vi "Main Tclk.vi"() -> ()   [LabVIEW 2018] (continued)
            n6787 = local read "Faraday Cup < Milling current"() -> (w2106:bool)
            n6788 = local read "FIB"() -> (w2105:bool)
            n6789 = local read "Email Alert Recipients"() -> (w2110:string[])
            n6790 = local read "Mail server"() -> (w2111:string)
            n6791 = local read "Hardware Configuration"() -> (w2113:T25)
            n6792 = local read "Email Log Files"() -> (w2108:path)
            n6793 = Unbundle By Name(w2113) -> ("Machine ID"=w2112:string)
            n6794 = Compound Arithmetic op=AND(w2105, w2106) -> (w2107:bool)
            n6795 = call "Email alert.vi"("Email log file path"=w2108, "Send email"=w2107, "Machine ID"=w2112, "Mail server"=w2111, "Alarm message"="Faraday cup current < Milling current", "Recipents"=w2110) -> ()  [unwired: 6 in]
            n6796 = case shown="True" w2107 {
              frame False {
              }
              frame True {
                n6797 = stacked-sequence {
                  frame #0 {
                    n6798 = Wait (ms)(milliseconds to wait=u32 200) -> ()  [unwired: 1 out]
                  }
                  frame #1 {
                    n6799 = local write "Faraday Cup < Milling current"(FALSE ("E-mail test")) -> ()
                  }
                }
              }
            }
          }
          frame #6 {
            n6800 = local read "SEM Status"() -> (w2122:T12)
            n6801 = Unbundle By Name(w2122) -> ("SEM Spec. I (nA)"=w2119:sgl)
            n6802 = local read "FIB"() -> (w2118:bool)
            n6803 = local read "SEM Spec. I spike"() -> (w2117:bool)
            n6804 = local read "Email Alert Recipients"() -> (w2127:string[])
            n6805 = local read "Mail server"() -> (w2128:string)
            n6806 = local read "Hardware Configuration"() -> (w2130:T25)
            n6807 = local read "Email Log Files"() -> (w2126:path)
            n6808 = Format Into String(format string="%#g", w2119) -> (resulting string=w2120:string)  [unwired: 2 in, 1 out]
            n6809 = Compound Arithmetic op=AND(w2118, w2117) -> (w2116:bool)
            n6810 = Unbundle By Name(w2130) -> ("Machine ID"=w2129:string)
            n6811 = Concatenate Strings("SEM specimen current spiked to " ("Alarm message"), w2120, " nA" ("Alarm message")) -> (w2124:string)
            n6812 = call "Email alert.vi"("Email log file path"=w2126, "Send email"=w2116, "Machine ID"=w2129, "Mail server"=w2128, "Alarm message"=w2124, "Recipents"=w2127) -> ()  [unwired: 6 in]
            n6813 = case shown="True" w2116 {
              frame False {
              }
              frame True {
                n6814 = stacked-sequence {
                  frame #0 {
                    n6815 = Wait (ms)(milliseconds to wait=u32 200) -> ()  [unwired: 1 out]
                  }
                  frame #1 {
                    n6816 = local write "SEM Spec. I spike"(FALSE ("E-mail test")) -> ()
                  }
                }
              }
            }
          }
          frame #7 {
            n6817 = local read "Milling Z voltage (V)"() -> (w2136:sgl)
            n6818 = local read "FIB"() -> (w2135:bool)
            n6819 = local read "Milling Z voltage spike"() -> (w2134:bool)
            n6820 = local read "Email Alert Recipients"() -> (w2143:string[])
            n6821 = local read "Mail server"() -> (w2144:string)
            n6822 = local read "Hardware Configuration"() -> (w2146:T25)
            n6823 = local read "Email Log Files"() -> (w2142:path)
            n6824 = Format Into String(format string="%#g", w2136) -> (resulting string=w2137:string)  [unwired: 2 in, 1 out]
            n6825 = Unbundle By Name(w2146) -> ("Machine ID"=w2145:string)
            n6826 = Compound Arithmetic op=AND(w2135, w2134) -> (w2133:bool)
            n6827 = Concatenate Strings("Milling Z voltage spiked to " ("Alarm message"), w2137, " V" ("Alarm message")) -> (w2140:string)
            n6828 = call "Email alert.vi"("Email log file path"=w2142, "Send email"=w2133, "Machine ID"=w2145, "Mail server"=w2144, "Alarm message"=w2140, "Recipents"=w2143) -> ()  [unwired: 6 in]
            n6829 = case shown="True" w2133 {
              frame False {
              }
              frame True {
                n6830 = stacked-sequence {
                  frame #0 {
                    n6831 = Wait (ms)(milliseconds to wait=u32 200) -> ()  [unwired: 1 out]
                  }
                  frame #1 {
                    n6832 = local write "Milling Z voltage spike"(FALSE ("E-mail test")) -> ()
                  }
                }
              }
            }
          }
          frame #8 {
            n6833 = local read "Alert Settings"() -> (w2153:T36)
            n6834 = local read "FIB"() -> (w2149:bool)
            n6835 = Unbundle By Name(w2153) -> ("EHT off alarm"=w2152:bool)
            n6836 = local read "EHT off"() -> (w2154:bool)
            n6837 = local read "Email Alert Recipients"() -> (w2156:string[])
            n6838 = local read "Mail server"() -> (w2157:string)
            n6839 = local read "Hardware Configuration"() -> (w2159:T25)
            n6840 = local read "Email Log Files"() -> (w2150:path)
            n6841 = Compound Arithmetic op=AND(w2149, w2152, w2154) -> (w2151:bool)
            n6842 = Unbundle By Name(w2159) -> ("Machine ID"=w2158:string)
            n6843 = call "Email alert.vi"("Email log file path"=w2150, "Send email"=w2151, "Machine ID"=w2158, "Mail server"=w2157, "Alarm message"="EHT was off", "Recipents"=w2156) -> ()  [unwired: 6 in]
            n6844 = case shown="True" w2151 {
              frame False {
              }
              frame True {
                n6845 = stacked-sequence {
                  frame #0 {
                    n6846 = Wait (ms)(milliseconds to wait=u32 200) -> ()  [unwired: 1 out]
                  }
                  frame #1 {
                    n6847 = local write "EHT off"(FALSE ("E-mail test")) -> ()
                  }
                }
              }
            }
          }
          frame #9 {
            n6848 = local read "Alert Settings"() -> (w2166:T36)
            n6849 = local read "FIB"() -> (w2162:bool)
            n6850 = local read "Det A over scale"() -> (w2164:bool)
            n6851 = local read "Email Alert Recipients"() -> (w2169:string[])
            n6852 = local read "Mail server"() -> (w2170:string)
            n6853 = local read "Hardware Configuration"() -> (w2172:T25)
            n6854 = local read "Email Log Files"() -> (w2167:path)
            n6855 = Unbundle By Name(w2166) -> ("Detector over scale warning"=w2165:bool)
            n6856 = Unbundle By Name(w2172) -> ("Machine ID"=w2171:string)
            n6857 = Compound Arithmetic op=AND(w2162, w2165, w2164) -> (w2163:bool)
            n6858 = call "Email alert.vi"("Email log file path"=w2167, "Send email"=w2163, "Machine ID"=w2171, "Mail server"=w2170, "Alarm message"="Detector A over scale", "Recipents"=w2169) -> ()  [unwired: 6 in]
            n6859 = case shown="True" w2163 {
              frame False {
              }
              frame True {
                n6860 = stacked-sequence {
                  frame #0 {
                    n6861 = Wait (ms)(milliseconds to wait=u32 200) -> ()  [unwired: 1 out]
                  }
                  frame #1 {
                    n6862 = local write "Det A over scale"(FALSE ("E-mail test")) -> ()
                  }
                }
              }
            }
          }
          frame #10 {
            n6863 = local read "Alert Settings"() -> (w2179:T36)
            n6864 = local read "FIB"() -> (w2175:bool)
            n6865 = local read "Email Alert Recipients"() -> (w2182:string[])
            n6866 = local read "Mail server"() -> (w2183:string)
            n6867 = local read "Hardware Configuration"() -> (w2185:T25)
            n6868 = local read "Email Log Files"() -> (w2180:path)
            n6869 = local read "Det B over scale"() -> (w2177:bool)
            n6870 = Unbundle By Name(w2179) -> ("Detector over scale warning"=w2178:bool)
            n6871 = Unbundle By Name(w2185) -> ("Machine ID"=w2184:string)
            n6872 = Compound Arithmetic op=AND(w2175, w2178, w2177) -> (w2176:bool)
            n6873 = call "Email alert.vi"("Email log file path"=w2180, "Send email"=w2176, "Machine ID"=w2184, "Mail server"=w2183, "Alarm message"="Detector B over scale", "Recipents"=w2182) -> ()  [unwired: 6 in]
            n6874 = case shown="True" w2176 {
              frame False {
              }
              frame True {
                n6875 = stacked-sequence {
                  frame #0 {
                    n6876 = Wait (ms)(milliseconds to wait=u32 200) -> ()  [unwired: 1 out]
                  }
                  frame #1 {
                    n6877 = local write "Det B over scale"(FALSE ("E-mail test")) -> ()
                  }
                }
              }
            }
          }
          frame #11 {
            n6878 = local read "Alert Settings"() -> (w2190:T36)
            n6879 = local read "3D image paused active"() -> (w2193:bool)
            n6880 = local read "3D image paused armed"() -> (w2191:bool)
            n6881 = local read "Hardware Configuration"() -> (w2198:T25)
            n6882 = local read "Email Log Files"() -> (w2188:path)
            n6883 = Unbundle By Name(w2190) -> ("3D imaging paused alarm"=w2189:bool)
            n6884 = Unbundle By Name(w2198) -> ("Machine ID"=w2194:string)
            n6885 = case shown="True" w2193 {
              frame False {
              }
              frame True {
                n6886 = stacked-sequence {
                  frame #0 {
                    n6887 = Wait (ms)(milliseconds to wait=u32 500) -> ()  [unwired: 1 out]
                  }
                  frame #1 {
                    w2200 = FALSE ("3D image paused active bypass")
                    n6888 = local write "3D image paused active"(w2200) -> ()
                    "3D image paused armed" <- w2200
                  }
                }
              }
            }
            n6889 = Compound Arithmetic op=AND(w2193, w2191, w2189) -> (w2192:bool)
            n6890 = call "Email alert.vi"("Email log file path"=w2188, "Send email"=w2192, "Machine ID"=w2194, "Mail server"="Mail server", "Alarm message"="3D imaging paused", "Recipents"="Email Alert Recipients") -> ()  [unwired: 6 in]
          }
          frame #12 {
            n6891 = local read "Alert Settings"() -> (w2206:T36)
            n6892 = local read "Email Alert Recipients"() -> (w2210:string[])
            n6893 = local read "API timeout"() -> (w2201:bool)
            n6894 = local read "SW error warning active"() -> (w2203:bool)
            n6895 = local read "SW error warning armed"() -> (w2207:bool)
            n6896 = local read "Mail server"() -> (w2211:string)
            n6897 = local read "Hardware Configuration"() -> (w2213:T25)
            n6898 = local read "Email Log Files"() -> (w2204:path)
            n6899 = Unbundle By Name(w2206) -> ("SW error warning"=w2205:bool)
            n6900 = Or(x=w2201, y=w2203) -> (x .or. y?=w2202:bool)
            n6901 = Unbundle By Name(w2213) -> ("Machine ID"=w2212:string)
            n6902 = Compound Arithmetic op=AND(w2202, w2207, w2205) -> (w2208:bool)
            n6903 = call "Email alert.vi"("Email log file path"=w2204, "Send email"=w2208, "Machine ID"=w2212, "Mail server"=w2211, "Alarm message"="Software timeout error", "Recipents"=w2210) -> ()  [unwired: 6 in]
            n6904 = case shown="True" w2202 {
              frame False {
              }
              frame True {
                n6905 = stacked-sequence {
                  frame #0 {
                    n6906 = Wait (ms)(milliseconds to wait=u32 500) -> ()  [unwired: 1 out]
                  }
                  frame #1 {
                    w2215 = FALSE ("3D image paused active bypass")
                    n6907 = local write "SW error warning active"(w2215) -> ()
                    "SW error warning armed" <- w2215
                  }
                }
              }
            }
          }
          frame #13 {
            n6908 = local read "SEM shutter failed active"() -> (w2224:bool)
            n6909 = local read "SEM shutter warning armed"() -> (w2225:bool)
            n6910 = local read "Email Alert Recipients"() -> (w2227:string[])
            n6911 = local read "Mail server"() -> (w2228:string)
            n6912 = local read "Hardware Configuration"() -> (w2230:T25)
            n6913 = local read "Email Log Files"() -> (w2223:path)
            n6914 = local read "Fail #"() -> (w2216:u8)
            n6915 = Greater Than 0?(x=w2216) -> (x > 0?=w2217:bool)
            n6916 = Format Into String(format string="%#g", w2216) -> (resulting string=w2220:string)  [unwired: 2 in, 1 out]
            n6917 = Concatenate Strings("SEM shutter failed " ("Alarm message"), w2220, " times" ("Alarm message")) -> (w2218:string)
            n6918 = Unbundle By Name(w2230) -> ("Machine ID"=w2229:string)
            n6919 = Compound Arithmetic op=AND(w2224, w2225, w2217) -> (w2226:bool)
            n6920 = call "Email alert.vi"("Email log file path"=w2223, "Send email"=w2226, "Machine ID"=w2229, "Mail server"=w2228, "Alarm message"=w2218, "Recipents"=w2227) -> ()  [unwired: 6 in]
            n6921 = case shown="True" w2224 {
              frame False {
              }
              frame True {
                n6922 = stacked-sequence {
                  frame #0 {
                    n6923 = Wait (ms)(milliseconds to wait=u32 500) -> ()  [unwired: 1 out]
                  }
                  frame #1 {
                    w2232 = FALSE ("3D image paused active bypass")
                    n6924 = local write "SEM shutter failed active"(w2232) -> ()
                    "SEM shutter warning armed" <- w2232
                  }
                }
              }
            }
          }
          frame #14 {
            n6925 = local read "Machine Type"() -> (w2233:u8)
            n6926 = case shown="2" w2233 {
              tunnel: [w2249 w2263] -> w2236
              frame 0, Default {
                w2244 = "%#g" ("format string")
                n6927 = local read "Actual Reheat Parameters"() -> (w2257:T1)
                n6928 = local read "HV Data Output"() -> (w2248:T18)
                n6929 = Unbundle By Name(w2248) -> ("Tip Lifetime (hr)"=w2247:sgl)
                n6930 = Unbundle By Name(w2257) -> ("Filament I (A)"=w2256:sgl, "Reheat time (s)"=w2255:sgl)
                n6931 = Format Into String(format string=w2244, w2256) -> (resulting string=w2253:string)  [unwired: 2 in, 1 out]
                n6932 = Format Into String(format string="%d", w2247) -> (resulting string=w2245:string)  [unwired: 2 in, 1 out]
                n6933 = Format Into String(format string=w2244, w2255) -> (resulting string=w2251:string)  [unwired: 2 in, 1 out]
                n6934 = Concatenate Strings("FIB lifetime = " ("Alarm message"), w2245, " hr, FIB reheat started, " ("Alarm message"), w2253, " A for " ("string"), w2251, " s" ("string")) -> (w2249:string)
              }
              frame 2 {
                n6935 = local read "Capella HV Data Output"() -> (w2262:T17)
                n6936 = Unbundle By Name(w2262) -> ("Tip Lifetime (uAhr)"=w2261:sgl)
                n6937 = Format Into String(format string="%d", w2261) -> (resulting string=w2259:string)  [unwired: 2 in, 1 out]
                n6938 = Concatenate Strings("FIB lifetime = " ("Alarm message"), w2259, " uAhr, FIB reheat started" ("Alarm message")) -> (w2263:string)
              }
            }
            n6939 = local read "Mail server"() -> (w2240:string)
            n6940 = local read "Hardware Configuration"() -> (w2242:T25)
            n6941 = local read "Send reheat start email"() -> (w2234:bool)
            n6942 = local read "Reheat warning armed"() -> (w2237:bool)
            n6943 = local read "Email Alert Recipients"() -> (w2239:string[])
            n6944 = Unbundle By Name(w2242) -> ("Machine ID"=w2241:string)
            n6945 = Compound Arithmetic op=AND(w2234, w2237) -> (w2238:bool)
            n6946 = local read "Email Log Files"() -> (w2235:path)
            n6947 = call "Email alert.vi"("Email log file path"=w2235, "Send email"=w2238, "Machine ID"=w2241, "Mail server"=w2240, "Alarm message"=w2236, "Recipents"=w2239) -> ()  [unwired: 6 in]
            n6948 = case shown="True" w2234 {
              frame False {
              }
              frame True {
                n6949 = stacked-sequence {
                  frame #0 {
                    n6950 = Wait (ms)(milliseconds to wait=u32 500) -> ()  [unwired: 1 out]
                  }
                  frame #1 {
                    w2266 = FALSE ("3D image paused active bypass")
                    n6951 = local write "Send reheat start email"(w2266) -> ()
                    "Reheat warning armed" <- w2266
                  }
                }
              }
            }
          }
          frame #15 {
            n6952 = local read "Start Reheat"() -> (w2278:bool)
            n6953 = local read "Reheat warning armed"() -> (w2277:bool)
            n6954 = local read "Reheat completed"() -> (w2274:bool)
            n6955 = local read "Machine Type"() -> (w2267:u8)
            n6956 = case shown="2" w2267 {
              tunnel: [w2297 w2319] -> w2271
              tunnel: [w2291 w2316] -> w2268
              frame 0, Default {
                w2283 = "%5.1f" ("format string")
                w2285 = "%#g" ("format string")
                n6957 = local read "Reheat Output"() -> (w2305:T21)
                n6958 = local read "HV Data Output"() -> (w2292:T18)
                n6959 = Unbundle By Name(w2305) -> ("Initial emission (uA)"=w2304:sgl, "Initial suppressor (V)"=w2303:sgl, "V/I Slope"=w2296:sgl, "Reheat Success"=w2291:bool)
                n6960 = Unbundle By Name(w2292) -> ("Suppressor (V)"=w2290:sgl, "Emission (uA)"=w2288:sgl)
                n6961 = Format Into String(format string=w2283, w2304) -> (resulting string=w2301:string)  [unwired: 2 in, 1 out]
                n6962 = Format Into String(format string=w2283, w2296) -> (resulting string=w2295:string)  [unwired: 2 in, 1 out]
                n6963 = Format Into String(format string=w2285, w2290) -> (resulting string=w2289:string)  [unwired: 2 in, 1 out]
                n6964 = Format Into String(format string=w2285, w2303) -> (resulting string=w2299:string)  [unwired: 2 in, 1 out]
                n6965 = Format Into String(format string="%3.1f", w2288) -> (resulting string=w2287:string)  [unwired: 2 in, 1 out]
                n6966 = Concatenate Strings("FIB reheat completed successfully, initial emission: " ("Alarm message"), w2301, " uA @ suppressor = " ("element"), w2299, " V, V/I slope = " ("element"), w2295, ", suppressor = " ("string"), w2289, " V @ " ("string"), w2287, " uA emission " ("string")) -> (w2297:string)
              }
              frame 2 {
                w2306 = "%3.1f" ("format string")
                n6967 = local read "Capella HV Data Output"() -> (w2317:T17)
                n6968 = local read "Reheat Output"() -> (w2320:T21)
                n6969 = Unbundle By Name(w2320) -> ("Reheat Success"=w2316:bool)
                n6970 = Unbundle By Name(w2317) -> ("Suppressor (V)"=w2315:sgl, "Emission Actual (uA)"=w2313:sgl)
                n6971 = local read "FIB V/I slope"() -> (w2308:sgl)
                n6972 = Format Into String(format string=w2306, w2308) -> (resulting string=w2307:string)  [unwired: 2 in, 1 out]
                n6973 = Format Into String(format string="%5.1f", w2315) -> (resulting string=w2314:string)  [unwired: 2 in, 1 out]
                n6974 = Format Into String(format string=w2306, w2313) -> (resulting string=w2312:string)  [unwired: 2 in, 1 out]
                n6975 = Concatenate Strings("FIB reheat completed successfully, suppressor =  " ("Alarm message"), w2314, " V @ " ("string"), w2312, " uA emission, V/I slope =  " ("string"), w2307) -> (w2319:string)
              }
            }
            n6976 = local read "Mail server"() -> (w2280:string)
            n6977 = local read "Hardware Configuration"() -> (w2282:T25)
            n6978 = Not(x=w2278) -> (.not. x?=w2275:bool)
            n6979 = Not(x=w2277) -> (.not. x?=w2276:bool)
            n6980 = Unbundle By Name(w2282) -> ("Machine ID"=w2281:string)
            n6981 = Compound Arithmetic op=AND(w2275, w2276, w2274) -> (w2279:bool)
            n6982 = local read "Email Alert Recipients"() -> (w2270:string[])
            n6983 = local read "Email Log Files"() -> (w2269:path)
            n6984 = case shown="True" w2275 {
              frame False {
              }
              frame True {
                n6985 = stacked-sequence {
                  frame #0 {
                    n6986 = Wait (ms)(milliseconds to wait=u32 500) -> ()  [unwired: 1 out]
                  }
                  frame #1 {
                    n6987 = local write "Reheat warning armed"(TRUE ("3D image paused active bypass")) -> ()
                  }
                }
              }
            }
            n6988 = Select(t=w2271, s=w2268, f="FIB reheat failed" ("Alarm message")) -> (s? t:f=w2273:string)
            n6989 = call "Email alert.vi"("Email log file path"=w2269, "Send email"=w2279, "Machine ID"=w2281, "Mail server"=w2280, "Alarm message"=w2273, "Recipents"=w2270) -> ()  [unwired: 6 in]
          }
          frame #16 {
            n6990 = local read "Email Alert Recipients"() -> (w2328:string[])
            n6991 = local read "Auto re-engage"() -> (w2324:bool)
            n6992 = local read "Re-engage warning armed"() -> (w2325:bool)
            n6993 = local read "Mail server"() -> (w2329:string)
            n6994 = local read "Hardware Configuration"() -> (w2331:T25)
            n6995 = local read "Email Log Files"() -> (w2323:path)
            n6996 = Unbundle By Name(w2331) -> ("Machine ID"=w2330:string)
            n6997 = Compound Arithmetic op=AND(w2324, w2325) -> (w2326:bool)
            n6998 = call "Email alert.vi"("Email log file path"=w2323, "Send email"=w2326, "Machine ID"=w2330, "Mail server"=w2329, "Alarm message"="Auto re-engaging started", "Recipents"=w2328) -> ()  [unwired: 6 in]
            n6999 = case shown="True" w2324 {
              frame False {
              }
              frame True {
                n7000 = stacked-sequence {
                  frame #0 {
                    n7001 = Wait (ms)(milliseconds to wait=u32 500) -> ()  [unwired: 1 out]
                  }
                  frame #1 {
                    "Re-engage warning armed" <- FALSE ("3D image paused active bypass")
                  }
                }
              }
            }
          }
          frame #17 {
            n7002 = local read "Email Alert Recipients"() -> (w2347:string[])
            n7003 = local read "Auto re-engage"() -> (w2339:bool)
            n7004 = local read "Re-engage warning armed"() -> (w2343:bool)
            n7005 = local read "Re-engage cancelled"() -> (w2335:bool)
            n7006 = local read "Re-engage counts"() -> (w2337:u8)
            n7007 = local read "Mail server"() -> (w2348:string)
            n7008 = local read "Hardware Configuration"() -> (w2350:T25)
            n7009 = local read "Email Log Files"() -> (w2340:path)
            n7010 = Not Equal?(x=w2338, y=w2337) -> (x != y?=w2336:bool)
            n7011 = Equal?(x=w2337, y=u8 50) -> (x = y?=w2341:bool)
            n7012 = Unbundle By Name(w2350) -> ("Machine ID"=w2349:string)
            n7013 = Not(x=w2343) -> (.not. x?=w2344:bool)
            n7014 = Not(x=w2335) -> (.not. x?=w2334:bool)
            n7015 = Compound Arithmetic op=AND(w2339, w2344, w2334, w2336, w2341) -> (w2345:bool)
            n7016 = call "Email alert.vi"("Email log file path"=w2340, "Send email"=w2345, "Machine ID"=w2349, "Mail server"=w2348, "Alarm message"="FI has not covered after 50 frames", "Recipents"=w2347) -> ()  [unwired: 6 in]
            n7017 = case shown="True" w2339 {
              frame False {
              }
              frame True {
                n7018 = stacked-sequence {
                  frame #0 {
                    n7019 = Wait (ms)(milliseconds to wait=u32 500) -> ()  [unwired: 1 out]
                  }
                  frame #1 {
                  }
                }
              }
            }
          }
          frame #18 {
            n7020 = local read "Email Alert Recipients"() -> (w2365:string[])
            n7021 = local read "Auto re-engage"() -> (w2357:bool)
            n7022 = local read "Re-engage warning armed"() -> (w2361:bool)
            n7023 = local read "Re-engage cancelled"() -> (w2353:bool)
            n7024 = local read "Re-engage counts"() -> (w2356:u8)
            n7025 = local read "Mail server"() -> (w2366:string)
            n7026 = local read "Hardware Configuration"() -> (w2368:T25)
            n7027 = local read "Email Log Files"() -> (w2358:path)
            n7028 = Not Equal?(x=w2355, y=w2356) -> (x != y?=w2354:bool)
            n7029 = Equal?(x=w2356, y=u8 100) -> (x = y?=w2359:bool)
            n7030 = Unbundle By Name(w2368) -> ("Machine ID"=w2367:string)
            n7031 = Not(x=w2361) -> (.not. x?=w2362:bool)
            n7032 = Not(x=w2353) -> (.not. x?=w2352:bool)
            n7033 = Compound Arithmetic op=AND(w2357, w2362, w2352, w2354, w2359) -> (w2363:bool)
            n7034 = call "Email alert.vi"("Email log file path"=w2358, "Send email"=w2363, "Machine ID"=w2367, "Mail server"=w2366, "Alarm message"="FI has not covered after 100 frames", "Recipents"=w2365) -> ()  [unwired: 6 in]
            n7035 = case shown="True" w2357 {
              frame False {
              }
              frame True {
                n7036 = stacked-sequence {
                  frame #0 {
                    n7037 = Wait (ms)(milliseconds to wait=u32 500) -> ()  [unwired: 1 out]
                  }
                  frame #1 {
                  }
                }
              }
            }
          }
          frame #19 {
            n7038 = local read "Email Alert Recipients"() -> (w2383:string[])
            n7039 = local read "Auto re-engage"() -> (w2375:bool)
            n7040 = local read "Re-engage warning armed"() -> (w2379:bool)
            n7041 = local read "Re-engage cancelled"() -> (w2371:bool)
            n7042 = local read "Re-engage counts"() -> (w2374:u8)
            n7043 = local read "Mail server"() -> (w2384:string)
            n7044 = local read "Hardware Configuration"() -> (w2386:T25)
            n7045 = local read "Email Log Files"() -> (w2376:path)
            n7046 = Not Equal?(x=w2373, y=w2374) -> (x != y?=w2372:bool)
            n7047 = Equal?(x=w2374, y=u8 200) -> (x = y?=w2377:bool)
            n7048 = Unbundle By Name(w2386) -> ("Machine ID"=w2385:string)
            n7049 = Not(x=w2379) -> (.not. x?=w2380:bool)
            n7050 = Not(x=w2371) -> (.not. x?=w2370:bool)
            n7051 = Compound Arithmetic op=AND(w2375, w2380, w2370, w2372, w2377) -> (w2381:bool)
            n7052 = call "Email alert.vi"("Email log file path"=w2376, "Send email"=w2381, "Machine ID"=w2385, "Mail server"=w2384, "Alarm message"="FI has not covered after 200 frames", "Recipents"=w2383) -> ()  [unwired: 6 in]
            n7053 = case shown="True" w2375 {
              frame False {
              }
              frame True {
                n7054 = stacked-sequence {
                  frame #0 {
                    n7055 = Wait (ms)(milliseconds to wait=u32 500) -> ()  [unwired: 1 out]
                  }
                  frame #1 {
                  }
                }
              }
            }
          }
          frame #20 {
            n7056 = local read "Auto re-engage"() -> (w2401:bool)
            n7057 = local read "Re-engage warning armed"() -> (w2399:bool)
            n7058 = local read "Re-engage cancelled"() -> (w2389:bool)
            n7059 = local read "Email Alert Recipients"() -> (w2403:string[])
            n7060 = local read "Re-engage counts"() -> (w2393:u8)
            n7061 = local read "Mail server"() -> (w2404:string)
            n7062 = local read "Hardware Configuration"() -> (w2406:T25)
            n7063 = local read "Email Log Files"() -> (w2398:path)
            n7064 = Not(x=w2401) -> (.not. x?=w2400:bool)
            n7065 = Subtract(x=w2393, y=u8 12) -> (x-y=w2392:u8)
            n7066 = Unbundle By Name(w2406) -> ("Machine ID"=w2405:string)
            n7067 = Not(x=w2399) -> (.not. x?=w2390:bool)
            n7068 = Not(x=w2389) -> (.not. x?=w2388:bool)
            n7069 = Format Into String(w2392) -> (resulting string=w2395:string)  [unwired: 3 in, 1 out]
            n7070 = Compound Arithmetic op=AND(w2400, w2390, w2388) -> (w2402:bool)
            n7071 = Concatenate Strings("Auto re-engaging finished, FI recovered in " ("Alarm message"), w2395, " frames" ("Alarm message")) -> (w2396:string)
            n7072 = call "Email alert.vi"("Email log file path"=w2398, "Send email"=w2402, "Machine ID"=w2405, "Mail server"=w2404, "Alarm message"=w2396, "Recipents"=w2403) -> ()  [unwired: 6 in]
            n7073 = case shown="True" w2400 {
              frame False {
              }
              frame True {
                n7074 = stacked-sequence {
                  frame #0 {
                    n7075 = Wait (ms)(milliseconds to wait=u32 500) -> ()  [unwired: 1 out]
                  }
                  frame #1 {
                    n7076 = local write "Re-engage warning armed"(TRUE ("3D image paused active bypass")) -> ()
                  }
                }
              }
            }
          }
          frame #21 {
            n7077 = local read "Auto re-engage"() -> (w2417:bool)
            n7078 = local read "Re-engage cancelled"() -> (w2409:bool)
            n7079 = local read "Email Alert Recipients"() -> (w2419:string[])
            n7080 = local read "Re-engage counts"() -> (w2410:u8)
            n7081 = local read "Mail server"() -> (w2420:string)
            n7082 = local read "Hardware Configuration"() -> (w2422:T25)
            n7083 = local read "Email Log Files"() -> (w2415:path)
            n7084 = Not(x=w2417) -> (.not. x?=w2416:bool)
            n7085 = Unbundle By Name(w2422) -> ("Machine ID"=w2421:string)
            n7086 = Format Into String(w2410) -> (resulting string=w2412:string)  [unwired: 3 in, 1 out]
            n7087 = Compound Arithmetic op=AND(w2416, w2409) -> (w2418:bool)
            n7088 = Concatenate Strings("Auto re-engaging cancelled after " ("Alarm message"), w2412, " frames" ("Alarm message")) -> (w2413:string)
            n7089 = call "Email alert.vi"("Email log file path"=w2415, "Send email"=w2418, "Machine ID"=w2421, "Mail server"=w2420, "Alarm message"=w2413, "Recipents"=w2419) -> ()  [unwired: 6 in]
            n7090 = case shown="True" w2416 {
              frame False {
              }
              frame True {
                n7091 = stacked-sequence {
                  frame #0 {
                    n7092 = Wait (ms)(milliseconds to wait=u32 500) -> ()  [unwired: 1 out]
                  }
                  frame #1 {
                    "Re-engage cancelled" <- FALSE ("3D image paused active bypass")
                  }
                }
              }
            }
          }
          frame #22 {
            w2426 = "%5.3f" ("format string")
            n7093 = local read "FIB"() -> (w2425:bool)
            n7094 = local read "Focus index warning active"() -> (w2430:bool)
            n7095 = local read "Alert Settings"() -> (w2434:T36)
            n7096 = local read "Email Alert Recipients"() -> (w2442:string[])
            n7097 = local read "Focus Index"() -> (w2427:sgl)
            n7098 = local read "Mail server"() -> (w2443:string)
            n7099 = local read "Hardware Configuration"() -> (w2445:T25)
            n7100 = local read "Focus index warning armed"() -> (w2440:bool)
            n7101 = Unbundle By Name(w2434) -> ("Focus index warning"=w2431:bool, "Focus index low limit"=w2433:sgl, "Run Auto Stig"=w2432:bool)
            n7102 = Unbundle By Name(w2445) -> ("Machine ID"=w2444:string)
            n7103 = Format Into String(format string=w2426, w2433) -> (resulting string=w2436:string)  [unwired: 2 in, 1 out]
            n7104 = Compound Arithmetic op=AND(w2425, w2430, w2440, w2431) -> (w2441:bool)
            n7105 = Format Into String(format string=w2426, w2427) -> (resulting string=w2439:string)  [unwired: 2 in, 1 out]
            n7106 = local read "Email Log Files"() -> (w2428:path)
            n7107 = Compound Arithmetic op=AND(w2430, w2431, w2432) -> (w2429:bool)
            n7108 = Concatenate Strings("Focus index dropped below " ("Alarm message"), w2436, " to " ("Alarm message"), w2439) -> (w2438:string)
            n7109 = call "Email alert.vi"("Email log file path"=w2428, "Send email"=w2441, "Machine ID"=w2444, "Mail server"=w2443, "Alarm message"=w2438, "Recipents"=w2442) -> ()  [unwired: 6 in]
            n7110 = case shown="True" w2430 {
              frame False {
              }
              frame True {
                n7111 = stacked-sequence {
                  frame #0 {
                    n7112 = Wait (ms)(milliseconds to wait=u32 500) -> ()  [unwired: 1 out]
                  }
                  frame #1 {
                    "Focus index warning armed" <- FALSE ("3D image paused active bypass")
                  }
                }
              }
            }
            n7113 = case shown="True" w2429 {
              frame False {
              }
              frame True {
                n7114 = local write "Auto Stig"(TRUE ("Auto Stig")) -> ()
              }
            }
          }
          frame #23 {
            w2453 = "%5.3f" ("format string")
            n7115 = local read "Focus index stop trigger active"() -> (w2458:bool)
            n7116 = local read "Alert Settings"() -> (w2461:T36)
            n7117 = local read "Email Alert Recipients"() -> (w2467:string[])
            n7118 = local read "Focus Index"() -> (w2454:sgl)
            n7119 = local read "Z removal stop threshold Z(nm)"() -> (w2449:u8)
            n7120 = local read "Mail server"() -> (w2468:string)
            n7121 = local read "Hardware Configuration"() -> (w2470:T25)
            n7122 = Unbundle By Name(w2461) -> ("Focus index warning"=w2459:bool, "Focus index stop limit"=w2460:sgl)
            n7123 = Unbundle By Name(w2470) -> ("Machine ID"=w2469:string)
            n7124 = Format Into String(format string=w2453, w2460) -> (resulting string=w2463:string)  [unwired: 2 in, 1 out]
            n7125 = Format Into String(format string=w2453, w2454) -> (resulting string=w2466:string)  [unwired: 2 in, 1 out]
            n7126 = Format Into String(format string="%d", w2449) -> (resulting string=w2451:string)  [unwired: 2 in, 1 out]
            n7127 = Compound Arithmetic op=AND(w2458, w2459) -> (w2455:bool)
            n7128 = local read "Email Log Files"() -> (w2457:path)
            n7129 = Concatenate Strings("Focus index dropped below " ("Alarm message"), w2463, " to " ("Alarm message"), w2466, " for " ("string"), w2451, "nm removal" ("string")) -> (w2465:string)
            n7130 = call "Email alert.vi"("Email log file path"=w2457, "Send email"=w2455, "Machine ID"=w2469, "Mail server"=w2468, "Alarm message"=w2465, "Recipents"=w2467) -> ()  [unwired: 6 in]
            n7131 = case shown="True" w2455 {
              frame False {
              }
              frame True {
                n7132 = stacked-sequence {
                  frame #0 {
                    n7133 = Wait (ms)(milliseconds to wait=u32 500) -> ()  [unwired: 1 out]
                  }
                  frame #1 {
                    n7134 = local write "Focus index stop trigger active"(FALSE ("Focus index stop trigger active")) -> ()
                    n7135 = local write "FI below limit counts"(u8 0 ("FI below limit counts")) -> ()
                  }
                }
              }
            }
          }
          frame #24 {
            n7136 = local read "Email Alert Recipients"() -> (w2486:string[])
            n7137 = local read "Focus index recovery active"() -> (w2483:bool)
            n7138 = local read "Focus index warning armed"() -> (w2484:bool)
            n7139 = local read "Alert Settings"() -> (w2478:T36)
            n7140 = local read "Focus Index"() -> (w2475:sgl)
            n7141 = local read "Mail server"() -> (w2487:string)
            n7142 = local read "Hardware Configuration"() -> (w2489:T25)
            n7143 = Unbundle By Name(w2478) -> ("Focus index warning"=w2477:bool)
            n7144 = Not(x=w2484) -> (.not. x?=w2479:bool)
            n7145 = Unbundle By Name(w2489) -> ("Machine ID"=w2488:string)
            n7146 = Compound Arithmetic op=AND(w2483, w2479, w2477) -> (w2485:bool)
            n7147 = Format Into String(format string="%5.3f", w2475) -> (resulting string=w2482:string)  [unwired: 2 in, 1 out]
            n7148 = local read "Email Log Files"() -> (w2476:path)
            n7149 = Concatenate Strings("Focus index recovered to " ("Alarm message"), w2482) -> (w2481:string)
            n7150 = call "Email alert.vi"("Email log file path"=w2476, "Send email"=w2485, "Machine ID"=w2488, "Mail server"=w2487, "Alarm message"=w2481, "Recipents"=w2486) -> ()  [unwired: 6 in]
            n7151 = case shown="True" w2483 {
              frame False {
              }
              frame True {
                n7152 = stacked-sequence {
                  frame #0 {
                    n7153 = Wait (ms)(milliseconds to wait=u32 500) -> ()  [unwired: 1 out]
                  }
                  frame #1 {
                    n7154 = local write "Focus index warning armed"(TRUE ("Focus index warning armed")) -> ()
                  }
                }
              }
            }
          }
          frame #25 {
            w2493 = "%5.3f" ("format string")
            n7155 = local read "Temp (F)"() -> (w2504:sgl)
            n7156 = local read "Temp range (F)"() -> (w2499:sgl)
            n7157 = local read "Temp gradient (F/min)"() -> (w2503:dbl)
            n7158 = local read "Mail server"() -> (w2512:string)
            n7159 = local read "Hardware Configuration"() -> (w2514:T25)
            n7160 = local read "Alert Settings"() -> (w2496:T36)
            n7161 = Format Into String(format string=w2493, w2504) -> (resulting string=w2508:string)  [unwired: 2 in, 1 out]
            n7162 = Format Into String(format string=w2493, w2499) -> (resulting string=w2497:string)  [unwired: 2 in, 1 out]
            n7163 = local read "Email Alert Recipients"() -> (w2511:string[])
            n7164 = local read "FIB"() -> (w2492:bool)
            n7165 = local read "Temperature warning active"() -> (w2502:bool)
            n7166 = local read "Temperature warning armed"() -> (w2501:bool)
            n7167 = Unbundle By Name(w2514) -> ("Machine ID"=w2513:string)
            n7168 = Format Into String(format string=w2493, w2503) -> (resulting string=w2506:string)  [unwired: 2 in, 1 out]
            n7169 = Unbundle By Name(w2496) -> ("Temperature alarm"=w2495:bool)
            n7170 = Concatenate Strings("Temperature reached " ("Alarm message"), w2508, " F, range @ " ("Alarm message"), w2497, " F, gradient @ " ("Alarm message"), w2506, " F/min" ("string")) -> (w2509:string)
            n7171 = local read "Email Log Files"() -> (w2494:path)
            n7172 = Compound Arithmetic op=AND(w2492, w2502, w2501, w2495) -> (w2500:bool)
            n7173 = call "Email alert.vi"("Email log file path"=w2494, "Send email"=w2500, "Machine ID"=w2513, "Mail server"=w2512, "Alarm message"=w2509, "Recipents"=w2511) -> ()  [unwired: 6 in]
            n7174 = case shown="True" w2502 {
              frame False {
              }
              frame True {
                n7175 = stacked-sequence {
                  frame #0 {
                    n7176 = Wait (ms)(milliseconds to wait=u32 500) -> ()  [unwired: 1 out]
                  }
                  frame #1 {
                    "Temperature warning armed" <- FALSE ("3D image paused active bypass")
                  }
                }
              }
            }
          }
          frame #26 {
            w2518 = "%5.3f" ("format string")
            n7177 = local read "Temp (F)"() -> (w2528:sgl)
            n7178 = local read "Temp range (F)"() -> (w2525:sgl)
            n7179 = local read "Temp gradient (F/min)"() -> (w2527:dbl)
            n7180 = local read "Mail server"() -> (w2536:string)
            n7181 = local read "Hardware Configuration"() -> (w2538:T25)
            n7182 = local read "Email Alert Recipients"() -> (w2535:string[])
            n7183 = local read "Alert Settings"() -> (w2521:T36)
            n7184 = Format Into String(format string=w2518, w2528) -> (resulting string=w2532:string)  [unwired: 2 in, 1 out]
            n7185 = Format Into String(format string=w2518, w2525) -> (resulting string=w2523:string)  [unwired: 2 in, 1 out]
            n7186 = local read "FIB"() -> (w2517:bool)
            n7187 = local read "Temperature recovery active"() -> (w2522:bool)
            n7188 = local read "Temperature warning armed"() -> (w2539:bool)
            n7189 = Format Into String(format string=w2518, w2527) -> (resulting string=w2530:string)  [unwired: 2 in, 1 out]
            n7190 = Unbundle By Name(w2521) -> ("Temperature alarm"=w2520:bool)
            n7191 = Unbundle By Name(w2538) -> ("Machine ID"=w2537:string)
            n7192 = Concatenate Strings("Temperature recovered to " ("Alarm message"), w2532, " F, range @ " ("Alarm message"), w2523, " F, gradient @ " ("Alarm message"), w2530, " F/min" ("string")) -> (w2533:string)
            n7193 = Not(x=w2539) -> (.not. x?=w2540:bool)
            n7194 = local read "Email Log Files"() -> (w2519:path)
            n7195 = Compound Arithmetic op=AND(w2517, w2522, w2540, w2520) -> (w2526:bool)
            n7196 = call "Email alert.vi"("Email log file path"=w2519, "Send email"=w2526, "Machine ID"=w2537, "Mail server"=w2536, "Alarm message"=w2533, "Recipents"=w2535) -> ()  [unwired: 6 in]
            n7197 = case shown="True" w2522 {
              frame False {
              }
              frame True {
                n7198 = stacked-sequence {
                  frame #0 {
                    n7199 = Wait (ms)(milliseconds to wait=u32 500) -> ()  [unwired: 1 out]
                  }
                  frame #1 {
                    n7200 = local write "Temperature warning armed"(TRUE ("Focus index warning armed")) -> ()
                  }
                }
              }
            }
          }
        }
        n7201 = Wait Until Next ms Multiple(millisecond multiple=u32 1000) -> ()  [unwired: 1 out]
        n7202 = local read "Stop"() -> (w1993:bool)
      }
      n7203 = Unregister For Events(event registration refnum=w712, error in=w713) -> (error out=w710:errorcluster)
      n7204 = Close Reference(reference=w714, error in (no error)=w710) -> ()  [unwired: 1 out]
      n7205 = while {
        stop <- w885 stop-if-true
        n7206 = local read "WatchDog Mode"() -> (w884:u16)
        n7207 = Wait Until Next ms Multiple(millisecond multiple=u32 1000) -> ()  [unwired: 1 out]
        n7208 = call "FM Gen Pulse for FIB-SEM.vi"("WatchDog Mode"=w884, "State Value"=i16 -2) -> ()  [unwired: 7 in, 3 out]
        n7209 = local read "Stop"() -> (w885:bool)
      }
      n7210 = while {
        stop <- w1329 stop-if-true
        n7211 = Wait Until Next ms Multiple(millisecond multiple=u32 100) -> ()  [unwired: 1 out]
        n7212 = case shown="True" "Load recipe" {
          frame False {
          }
          frame True {
            n7213 = stacked-sequence {
              frame #0 {
                n7214 = call "Recipe read write.vi"("Write"=FALSE, "Recipe path"="Read recipe path") -> ("Read output"=w1332:T119)  [unwired: 6 in, 3 out]
                n7215 = local read "Milling para"() -> (w1346:T35)
                n7216 = local read "FIB"() -> (w1357:bool)
                n7217 = Unbundle By Name(w1332) -> ("SEM Scan Parameters"=w1347:T5, "Detector Information"=w1348:T8, "SEM Options"=w1349:T27, "Focus Index Options"=w1331:T28, "Image fit to"=w1336:u8, "File Information"=w1350:T31, "Low mag SEM"=w1351:T30, "Mid Mag SEM"=w1340:T120, "FIB-SEM Angle"=w1352:dbl, "Milling para"=w1353:T35, "FI Detector"=w1358:u16, "Auto Optimzation"=w1359:bool, "Images per Auto Optimization"=w1360:u16, "AF Range (nm)"=w1361:sgl, "AF Steps"=w1362:u8, "AS Range (%)"=w1363:sgl, "AS Steps"=w1364:u8, "AA Range (%)"=w1338:sgl, "AA Steps"=w1337:u8, "X shift (nm/frame)"=w1355:dbl, "Y shift (nm/frame)"=w1354:dbl, "FIB Y zoom pixel (nm)"=w1356:dbl, "Mail server"=w1365:string, "Email Alert Recipients"=w1366:string[], "Alert Settings"=w1339:T121, "Reheat Parameters"=w1335:T1, "Start FIB HV DataLog"=w1334:bool, "Interval (s)"=w1333:u16)
                n7218 = local write "Recipe input"(w1332) -> ()
                n7219 = Not(x=w1357) -> (.not. x?=w1344:bool)
                n7220 = Unbundle By Name(w1346) -> ("Mill start from Last"=w1345:bool)
                n7221 = local write "Focus Index Options"(w1331) -> ()
                n7222 = local write "Image fit to"(w1336) -> ()
                n7223 = local write "FI Detector"(w1358) -> ()
                n7224 = local write "Auto Optimzation"(w1359) -> ()
                n7225 = local write "Images per Auto Optimization"(w1360) -> ()
                n7226 = local write "AF Range (nm)"(w1361) -> ()
                n7227 = local write "AF Steps"(w1362) -> ()
                n7228 = local write "AS Range (%)"(w1363) -> ()
                n7229 = local write "AS Steps"(w1364) -> ()
                n7230 = local write "AA Range (%)"(w1338) -> ()
                n7231 = local write "AA Steps"(w1337) -> ()
                n7232 = local write "Alert Settings"(w1339) -> ()
                n7233 = local write "Reheat Parameters"(w1335) -> ()
                n7234 = local write "Start FIB HV DataLog"(w1334) -> ()
                n7235 = local write "Interval (s)"(w1333) -> ()
                n7236 = Or(x=w1345, y=w1344) -> (x .or. y?=w1343:bool)
                n7237 = case shown="True" w1343 {
                  tunnel: w1347 -> [w1370 w1427]
                  tunnel: w1348 -> [_ w1413]
                  tunnel: w1349 -> [_ w1426]
                  tunnel: w1350 -> [_ w1425]
                  tunnel: w1351 -> [w1369 w1424]
                  tunnel: w1352 -> [_ w1423]
                  tunnel: w1353 -> [w1368 w1422]
                  tunnel: w1354 -> [_ w1421]
                  tunnel: w1355 -> [_ w1420]
                  tunnel: w1356 -> [_ w1419]
                  tunnel: w1365 -> [_ w1418]
                  tunnel: w1366 -> [_ w1417]
                  tunnel: w1340 -> [w1367 w1416]
                  frame False {
                    n7238 = stacked-sequence {
                      tunnel: w1370 -> [w1381 _ _]
                      tunnel: w1369 -> [_ w1401 _]
                      tunnel: w1368 -> [_ _ w1407]
                      tunnel: w1367 -> [_ w1393 _]
                      frame #0 {
                        n7239 = Unbundle By Name(w1381) -> ("X size (um)"=w1380:sgl, "Y size (um)"=w1379:sgl, "X size (V)"=w1378:dbl, "X size auto"=w1377:bool, "Scan rate (Hz)"=w1376:u32, "Oversampling"=w1375:u32, "Oversampling auto"=w1374:bool, "Frame line rampdown ratio"=w1373:sgl, "Pixel size (nm)"=w1372:sgl)
                        n7240 = local read "SEM Scan Parameters"() -> (w1382:T26)
                        n7241 = Bundle By Name(cluster=w1382, "X size (um)"=w1380, "Y size (um)"=w1379, "X size (V)"=w1378, "X size auto"=w1377, "Scan rate (Hz)"=w1376, "Oversampling"=w1375, "Oversampling auto"=w1374, "Frame line rampdown ratio"=w1373, "Pixel size (nm)"=w1372) -> (w1371:T26)
                        n7242 = local write "SEM Scan Parameters"(w1371) -> ()
                      }
                      frame #1 {
                        n7243 = Unbundle By Name(w1401) -> ("Low mag scan"=w1398:bool, "Prior to main scan"=w1397:bool, "Low mag interval"=w1396:u32, "Low mag scan rate (Hz)"=w1395:u32, "Show HM box"=w1394:bool)
                        n7244 = Unbundle By Name(w1393) -> ("Mid mag scan"=w1390:bool, "Prior to main scan"=w1389:bool, "Mid mag interval"=w1388:u32, "X size (um)"=w1387:sgl, "Y size (um)"=w1386:sgl, "Mid mag scan rate (Hz)"=w1385:u32, "Pixel size (nm)"=w1384:dbl, "Show MM box"=w1383:bool)
                        n7245 = local read "Mid Mag SEM"() -> (w1391:T29)
                        n7246 = Bundle By Name(cluster=w1391, "Mid mag scan"=w1390, "Prior to main scan"=w1389, "Mid mag interval"=w1388, "X size (um)"=w1387, "Y size (um)"=w1386, "Mid mag scan rate (Hz)"=w1385, "Pixel size (nm)"=w1384, "Show MM box"=w1383) -> (w1392:T29)
                        n7247 = local read "Low Mag SEM"() -> (w1400:T30)
